vi "PH_ImageOperator.constructor.vi"(0 "name":string, 2 "data in":string, 5 "error in (no error)":errorcluster) -> (14 "i ref out":refnum<vi>, 16 "data out":string, 19 "error out":errorcluster)   [LabVIEW 2014, in "PH_ImageOperator.lvlib"]
doc: "This class is forseen to operate on an image: it calculates several beam profile values. This class is connected to the class PH_ImageCalibrator which has to be used to produce a background image.\n\nThis class is part of the PHELIX user layer.\n\nauthor: Stefan Götte, GSI\n\nLicense Agreement for this software:\n\nCopyright (C)\nGesellschaft für Schwerionenforschung, GSI\nPlanckstr. 1\n64291 Darmstadt\nGermany\n\nContact: D.Beck@gsi.de \n\nThis program is free software; you can redistribute it and/or modify it under the terms of the \nGNU General Public License as published by the Free Software Foundation; either version 2 of \nthe license, or (at your option) any later version.\n\nThis program is distributed in the hope that it will be useful, but WITHOUT ANY WARRANTY; \nwithout even the implied warranty of MERCHANTABILITY or FITNESS FOR A PARTICULAR PURPOSE. See the GNU General License for more details (http://www.gnu.org).\n\nGesellschaft für Schwerionenforschung, GSI\nPlanckstr. 1, 64291 Darmstadt, Germany\nFor all questions and ideas contact: M.Richter@gsi.de, H.Brand@gsi.de or D.Beck@gsi.de.\nLast update: 16-JUN-2004"
uses:
  PH_ImageOperator.lvlib
  PH_ImageStatistician/PH_ImageStatistician.Statistician Data.ctl
  PH_ImageOperator.i attribute.ctl
  PH_StatusHandler/PH_StatusHandler.Status.ctl
  PH_ImageCalibrator/PH_ImageCalibrator.Calibration Data.ctl
  PH_ImageOperator.Beam Analysis Data.ctl
  <vilib>/vision/Image Controls.llb/IMAQ Image.ctl
  CSCore/BaseProcess/BaseProcess.lvlib
  PH_PSDBWriter/PH_PSDBWriter.lvlib
  PH_Common/PH_Common.lvlib
  PH_Img_BaseClass/PH_Img_BaseClass.lvlib
  PH_ImageStatistician/PH_ImageStatistician.lvlib
  PH_ImageCalibrator/PH_ImageCalibrator.lvlib
  PH_Class/PH_Class.lvlib
  PH_StatusHandler/PH_StatusHandler.lvlib
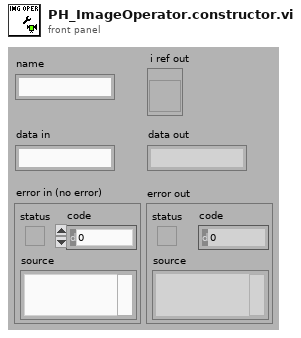
[diagram p1: front panel]
types:
  T1 = typedef "PH_ImageOperator.lvlib/PH_ImageOperator.i attribute.ctl" = cluster{"GUI Refs":cluster{"Delete":refnum<vi>, "Calibration status":refnum<vi>, "BI subtracted":refnum<vi>, "calc Energy":refnum<vi>, "Energy: expected value":refnum<vi>, "Energy: Tolerance":refnum<vi>, "Energy calculated":refnum<vi>, "Energy":refnum<vi>, "calc Beam Anal":refnum<vi>, "Maj Diam 1/esquare":refnum<vi>, "Min Diam 1/esquare":refnum<vi>, "Azi Angle":refnum<vi>, "Min/Maj Diam esquare":refnum<vi>, "Beam analysed":refnum<vi>, "CoG - x":refnum<vi>, "CoG - y":refnum<vi>, "BA: Method":refnum<vi>, "BA: Steps":refnum<vi>, "BA: Factor":refnum<vi>, "calc Traces":refnum<vi>, "Traces: Fit Gauss":refnum<vi>, "Traces calculated":refnum<vi>, "Maj FWHM":refnum<vi>, "Min FWHM":refnum<vi>, "Major Trace":refnum<vi>, "Minor Trace":refnum<vi>, "Maj Fit Order":refnum<vi>, "Min Fit Order":refnum<vi>, "Position calculated":refnum<vi>, "Position":refnum<vi>, "Type":refnum<vi>, "Center":refnum<vi>, "exp - X":refnum<vi>, "exp - Y":refnum<vi>, "Tolerance":refnum<vi>, "f":refnum<vi>, "M":refnum<vi>, "D":refnum<vi>, "q":refnum<vi>, "Dummy Method":refnum<vi>, "Dummy Type":refnum<vi>, "Global On":refnum<vi>, "Traces: No offset":refnum<vi>, "Maj 99%":refnum<vi>, "Min 99%":refnum<vi>, "GUI FF Image":refnum<vi>, "calc Fill Factor":refnum<vi>, "FF calculated":refnum<vi>, "Fill Factor: Filter?":refnum<vi>, "FF: Damage Threshold":refnum<vi>, "FF: Threshold":refnum<vi>, "FF: max allow. Energy":refnum<vi>, "FF: Fillfactor":refnum<vi>, "Calibration data":refnum<vi>}, "List of GUIs":string[], "Calibration":cluster{"Status":T2, "Calibration data":T3, "Calibration Data File":path}, "Final Image":cluster{"BI Subtraction Failure":bool}, "Energy":cluster{"on":bool, "expected value [mJ]":dbl, "Tolerance [%]":dbl, "State":T2, "Energy [mJ]":dbl, "Unit":string, "calculated @":timestamp}, "Beam Analysis":cluster{"on":bool, "Data":T4, "Method":bool, "Steps":i32, "Factor":i32, "ROI":cluster{"Left":i32, "Top":i32, "Right":i32, "Bottom":i32}, "analysed @":timestamp}, "Trace Analysis":cluster{"on":bool, "Fit on":bool, "Maj FWHM":dbl, "Min FWHM":dbl, "Maj Fit Order":i32, "Min Fit Order":i32, "No Offset":bool, "Maj 99%":dbl, "Min 99%":dbl, "Traces":cluster{"XScaleName":string, "Y Scale Minimum":sgl, "Y Scale Maximum":sgl, "X Scale Minimum":sgl, "X Scale Maximum":sgl, "Traces":cluster{"Index":sgl[], "Trace":dbl[]}[]}[], "analysed @":timestamp}, "Position Analysis":cluster{"on":bool, "exp - X":i32, "exp - Y":i32, "focal length [mm]":dbl, "Magnification":dbl, "Delta":dbl, "Theta":dbl, "Tolerance":dbl, "Type":bool, "analysed @":timestamp}, "Fill Factor":cluster{"on":bool, "Filter on?":bool, "Threshold":dbl, "Damage Threshold [J/cm²]":dbl, "Fillfactor":dbl, "Max. allowed Energy [J]":dbl, "calculated @":timestamp}, "Statistician Service ID":i32, "Images":cluster{"Background":T5, "OP":T5, "GUI":T5, "BA: ROI":T5, "Trace: Turn":T5, "FF: Main":T5, "FF: Help":T5, "PSDB: BG":T5, "PSDB: OP":T5, "PSDB: FF":T5}}
  T2 = typedef "PH_StatusHandler.lvlib/PH_StatusHandler.Status.ctl" = i16
  T3 = typedef "PH_ImageCalibrator.lvlib/PH_ImageCalibrator.Calibration Data.ctl" = cluster{"Date":string, "Time":string, "Cam Settings":cluster{"Cam ID":string, "Gain":dbl, "Brightness":dbl, "Shutter":dbl, "Cam Error":bool, "Mode":i32}, "Background Image":cluster{"Image":dbl[][], "Image Error":bool}, "Linear Calibration":cluster{"Calibration Factor":dbl, "not mm or mrad":bool}, "Energy Calibration":cluster{"Calibration Factor":dbl, "no mJ":bool}}
  T4 = typedef "PH_ImageOperator.lvlib/PH_ImageOperator.Beam Analysis Data.ctl" = cluster{"CoG-x":sgl, "CoG-y":sgl, "Maj Dim":dbl, "Min Dim":dbl, "Ellipticity":dbl, "Azimuth Angle [rad]":dbl, "Azi Angle rel to Maj?":bool}
  T5 = typedef "IMAQ Image.ctl" = refnum<image>
  T6 = typedef "PH_ImageStatistician.lvlib/PH_ImageStatistician.Statistician Data.ctl" = cluster{"Snapshot Time":dbl, "Maj FWHM":dbl, "Min FWHM":dbl, "Maj Fit Order":dbl, "Min Fit Order":dbl, "99% Diam Maj Trace":dbl, "99% Diam Min Trace":dbl, "Theta":dbl, "Delta":dbl, "Maj Diam":dbl, "Min Diam":dbl, "Azimuth Angle":dbl, "Azi Angle rel to major?":dbl, "Ellipticity":dbl, "CoG - X":dbl, "CoG - Y":dbl, "Energy":dbl, "Energy Cal - no mJ":dbl, "Lin Cal - no mm or mrad":dbl, "Lin Cal Factor":dbl}
  T7 = enum16{"SetAttribute", "GetAttribute", "CreateAttribute", "DestroyAttribute", "DestroyAllAtributes"}
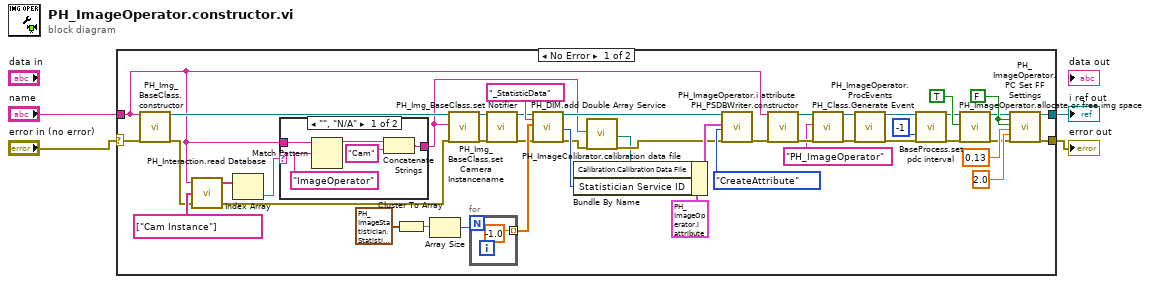
[diagram p0: block diagram]
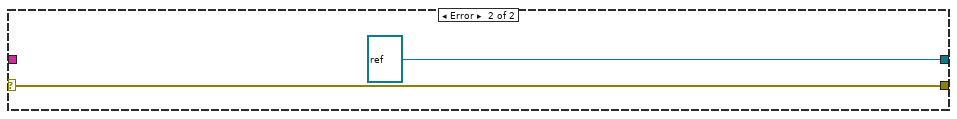
[diagram p3: hidden frame]
diagram:
  n1 = case shown="No Error" "error in (no error)" {
    selector: "error in (no error)" -> [w46 w57]
    tunnel: [w18 refnum<vi> refnum ("i ref out")] -> w4
    tunnel: [w17 w57] -> w3
    tunnel: "name" -> [w5 _]
    frame No Error {
      w43 = FALSE ("Calc Fill Factor")
      n2 = call "PH_Img_BaseClass.constructor.vi"("name"=w5, "error in(no error)"=w46) -> ("i ref out"=w9:refnum<vi>, "error out"=w10:errorcluster)  [unwired: 15 in, 1 out]
      n3 = call "PH_Interaction.read Database.vi"("error in (no error)"=w10, "Strings to search for"=string[] ["Cam Instance"], "DB Entry to read"=w5) -> ("error out"=w8:errorcluster, "Values"=w11:string[])  [unwired: 1 in]
      n4 = Index Array(array=w11) -> (element=w7:string)  [unwired: 1 in]
      n5 = case shown="\"\", \"N/A\"" w7 {
        selector: w7 -> [_ w55]
        tunnel: [w50 w55] -> w6
        tunnel: w5 -> [w54 _]
        frame "", "N/A" {
          n6 = Match Pattern(string=w54, regular expression="ImageOperator") -> (before substring=w52:string)  [unwired: 1 in, 3 out]
          n7 = Concatenate Strings(w52, "Cam" ("string")) -> (w50:string)
        }
        frame Default {
        }
      }
      n8 = Cluster To Array(cluster=T6 {"Snapshot Time"=0.0, "Maj FWHM"=0.0, "Min FWHM"=0.0, "Maj Fit Order"=0.0, "Min Fit Order"=0.0, "99% Diam Maj Trace"=0.0, "99% Diam Min Trace"=0.0, "Theta"=0.0, "Delta"=0.0, "Maj Diam"=0.0, "Min Diam"=0.0, "Azimuth Angle"=0.0, "Azi Angle rel to major?"=0.0, "Ellipticity"=0.0, "CoG - X"=0.0, "CoG - Y"=0.0, "Energy"=0.0, "Energy Cal - no mJ"=0.0, "Lin Cal - no mm or mrad"=0.0, "Lin Cal Factor"=0.0} ("Statistician Data")) -> (array=w36:dbl[])
      n9 = Array Size(array=w36) -> (size(s)=w39:i32)
      n10 = call "PH_Img_BaseClass.set Camera Instancename.vi"("i ref in"=w9, "Camera Instancename"=w6, "error in (no error)"=w8) -> ("i ref out"=w22:refnum<vi>, "error out"=w21:errorcluster)  [unwired: 15 in]
      n11 = for {
        N: w39 -> [_]
        tunnel: [-1.0] -> w38 mode=indexing
      }
      n12 = call "PH_Img_BaseClass.set Notifier.vi"("i ref in"=w22, "error in"=w21) -> ("i ref out"=w19:refnum<vi>, "error out"=w20:errorcluster)  [unwired: 16 in]
      n13 = call "PH_DIM.add Double Array Service.vi"("i ref in"=w19, "Service Name"="_StatisticData", "Double Value Array"=w38, "error in (no error)"=w20) -> ("i ref out"=w29:refnum<vi>, "Service ID"=w28:i32, "error out"=w16:errorcluster)  [unwired: 13 in]
      n14 = call "PH_ImageCalibrator.calibration data file.vi"("Camera Instance"=w6, "error in"=w16) -> ("File to save Cam Calibration Data in"=w14:path, "error out"=w15:errorcluster)  [unwired: 16 in]
      n15 = Bundle By Name(cluster=T1 {"GUI Refs"={"Delete"=refnum, "Calibration status"=refnum, "BI subtracted"=refnum, "calc Energy"=refnum, "Energy: expected value"=refnum, "Energy: Tolerance"=refnum, "Energy calculated"=refnum, "Energy"=refnum, "calc Beam Anal"=refnum, "Maj Diam 1/esquare"=refnum, "Min Diam 1/esquare"=refnum, "Azi Angle"=refnum, "Min/Maj Diam esquare"=refnum, "Beam analysed"=refnum, "CoG - x"=refnum, "CoG - y"=refnum, "BA: Method"=refnum, "BA: Steps"=refnum, "BA: Factor"=refnum, "calc Traces"=refnum, "Traces: Fit Gauss"=refnum, "Traces calculated"=refnum, "Maj FWHM"=refnum, "Min FWHM"=refnum, "Major Trace"=refnum, "Minor Trace"=refnum, "Maj Fit Order"=refnum, "Min Fit Order"=refnum, "Position calculated"=refnum, "Position"=refnum, "Type"=refnum, "Center"=refnum, "exp - X"=refnum, "exp - Y"=refnum, "Tolerance"=refnum, "f"=refnum, "M"=refnum, "D"=refnum, "q"=refnum, "Dummy Method"=refnum, "Dummy Type"=refnum, "Global On"=refnum, "Traces: No offset"=refnum, "Maj 99%"=refnum, "Min 99%"=refnum, "GUI FF Image"=refnum, "calc Fill Factor"=refnum, "FF calculated"=refnum, "Fill Factor: Filter?"=refnum, "FF: Damage Threshold"=refnum, "FF: Threshold"=refnum, "FF: max allow. Energy"=refnum, "FF: Fillfactor"=refnum, "Calibration data"=refnum}, "List of GUIs"=[], "Calibration"={"Status"=0, "Calibration data"={"Date"="", "Time"="", "Cam Settings"={"Cam ID"="", "Gain"=0.0, "Brightness"=0.0, "Shutter"=0.0, "Cam Error"=FALSE, "Mode"=0}, "Background Image"={"Image"=[], "Image Error"=FALSE}, "Linear Calibration"={"Calibration Factor"=0.0, "not mm or mrad"=FALSE}, "Energy Calibration"={"Calibration Factor"=0.0, "no mJ"=FALSE}}, "Calibration Data File"=path ""}, "Final Image"={"BI Subtraction Failure"=FALSE}, "Energy"={"on"=FALSE, "expected value [mJ]"=0.0, "Tolerance [%]"=0.0, "State"=0, "Energy [mJ]"=0.0, "Unit"="", "calculated @"=timestamp(0 s since 1904-01-01)}, "Beam Analysis"={"on"=FALSE, "Data"={"CoG-x"=0.0, "CoG-y"=0.0, "Maj Dim"=0.0, "Min Dim"=0.0, "Ellipticity"=0.0, "Azimuth Angle [rad]"=0.0, "Azi Angle rel to Maj?"=FALSE}, "Method"=FALSE, "Steps"=3, "Factor"=3, "ROI"={"Left"=0, "Top"=0, "Right"=0, "Bottom"=0}, "analysed @"=timestamp(0 s since 1904-01-01)}, "Trace Analysis"={"on"=FALSE, "Fit on"=FALSE, "Maj FWHM"=0.0, "Min FWHM"=0.0, "Maj Fit Order"=0, "Min Fit Order"=0, "No Offset"=FALSE, "Maj 99%"=0.0, "Min 99%"=0.0, "Traces"=[], "analysed @"=timestamp(0 s since 1904-01-01)}, "Position Analysis"={"on"=FALSE, "exp - X"=0, "exp - Y"=0, "focal length [mm]"=0.0, "Magnification"=0.0, "Delta"=0.0, "Theta"=0.0, "Tolerance"=0.0, "Type"=FALSE, "analysed @"=timestamp(0 s since 1904-01-01)}, "Fill Factor"={"on"=FALSE, "Filter on?"=FALSE, "Threshold"=0.0, "Damage Threshold [J/cm²]"=0.0, "Fillfactor"=0.0, "Max. allowed Energy [J]"=0.0, "calculated @"=timestamp(0 s since 1904-01-01)}, "Statistician Service ID"=0, "Images"={"Background"=refnum, "OP"=refnum, "GUI"=refnum, "BA: ROI"=refnum, "Trace: Turn"=refnum, "FF: Main"=refnum, "FF: Help"=refnum, "PSDB: BG"=refnum, "PSDB: OP"=refnum, "PSDB: FF"=refnum}} ("CLASS.i attribute"), "Calibration.Calibration Data File"=w14, "Statistician Service ID"=w28) -> (w34:T1)
      n16 = call "PH_ImageOperator.i attribute.vi"("VI Refnum"=w29, "CLASS.i attribute"=w34, "Action"=T7."CreateAttribute", "error in (no error)"=w15) -> ("error out"=w13:errorcluster)  [unwired: 13 in, 2 out]
      n17 = call "PH_PSDBWriter.constructor.vi"("name"=w5, "error in"=w13) -> ("i ref out"=w33:refnum<vi>, "error out"=w32:errorcluster)  [unwired: 15 in, 1 out]
      n18 = call "PH_Class.Generate Event.vi"("i ref in"=w33, "Class"="PH_ImageOperator", "error in (no error)"=w32) -> ("i ref out"=w31:refnum<vi>, "error out"=w30:errorcluster)  [unwired: 15 in]
      n19 = call "PH_ImageOperator.ProcEvents.vi"("i ref in"=w31, "error in (no error)"=w30) -> ("i ref out"=w27:refnum<vi>, "error out"=w26:errorcluster)  [unwired: 16 in]
      n20 = call "BaseProcess.set pdc interval.vi"("i ref in"=w27, "PeriodicInterval [ms]"=-1 ("PeriodicInterval"), "error in (no error)"=w26) -> ("i ref out"=w45:refnum<vi>, "error out"=w44:errorcluster)  [unwired: 14 in, 1 out]
      n21 = call "PH_ImageOperator.allocate or free img space.vi"("i ref in"=w45, "Allocate?"=TRUE, "error in (no error)"=w44) -> ("i ref out"=w24:refnum<vi>, "error out"=w23:errorcluster)  [unwired: 15 in]
      n22 = call "PH_ImageOperator.PC Set FF Settings.vi"("i ref in"=w24, "Calc Fill Factor"=w43, "Filter"=w43, "Threshold"=0.13, "Damage Threshold [J/cm²]"=2.0, "error in (no error)"=w23) -> ("i ref out"=w18:refnum<vi>, "error out"=w17:errorcluster)  [unwired: 12 in]
    }
    frame Error {
    }
  }
  "i ref out" <- w4
  "error out" <- w3
